vi "lfw_pairs.vi"(8 "error in (no error)":errorcluster caption="entrée d'erreur (pas d'erreur)", 11 "fetch_lfw_pairs":T2={"subset"="train", "funneled"=TRUE, "resize"=0.5, "color"=FALSE, "slice_"={"Cluster"={"height"=70, "width"=195}, "Cluster 2"={"height"=78, "width"=172}}, "download_if_missing"=TRUE, "Returns"="Data"}) -> (0 "error out":errorcluster, 3 "Data":T1)   [LabVIEW 2020]
doc: "Parameters :\n\n- subset : optional, default: ‘train’\nSelect the dataset to load: ‘train’ for the development training set, ‘test’ for the development test set, and ‘10_folds’ for the official evaluation set that is meant to be used with a 10-folds cross validation.\n\n- funneled : boolean, optional, default: True\nDownload and use the funneled variant of the dataset.\n\n- resize : float, optional, default 0.5\nRatio used to resize the each face picture.\n\n- color : boolean, optional, default False\nKeep the 3 RGB channels instead of averaging them to a single gray level channel. If color is True the shape of the data has one more dimension than the shape with color = False.\n\n- slice_ : optional\nProvide a custom 2D slice (height, width) to extract the ‘interesting’ part of the jpeg files and avoid use statistical correlation from the background\n\n- download_if_missing : optional, True by default\nIf False, raise a IOError if the data is not locally available instead of trying to download the data from the source site.\n\nReturns :\n\n- data : ndarray of shape (2200, 2, 62, 47). Shape depends on subset\nEach row has 2 face images corresponding to same or different person from the dataset containing 5749 people. Changing the slice_, resize or subset parameters will change the shape of the output.\n\n- target : numpy array of shape (2200,). Shape depends on subset.\nLabels associated to each pair of images. The two label values being different persons or the same person.\n\n\nEach picture is centered on a single face. The typical task is called Face Verification: given a pair of two pictures, a binary classifier must predict whether the two images are from the same person.\n\nBoth Face Verification and Face Recognition are tasks that are typically performed on the output of a model trained to perform Face Detection. The most popular model for Face Detection is called Viola-Jones and is implemented in the OpenCV library. The LFW faces were extracted by this face detector from various online websites.\n\nThe original images are 250 x 250 pixels, but the default slice and resize arguments reduce them to 62 x 47."
uses:
  lfw_pairs.lvclass
panel:
  out "lfw_pairs.lvclass":refnum<class "lfw_pairs.lvclass">
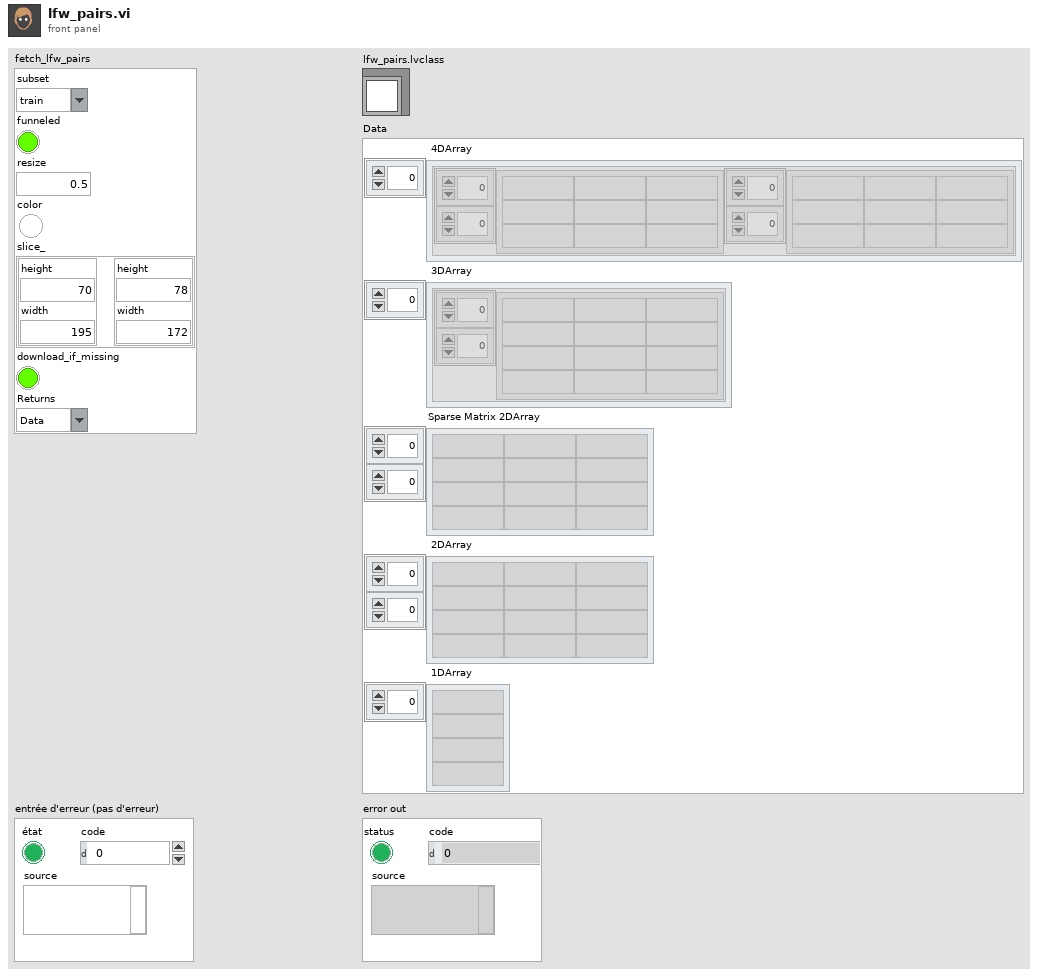
[diagram p1: front panel]
types:
  T1 = cluster{" 4DArray":cluster{"1":string[][], "2":string[][]}[], " 3DArray":cluster{"Tableau":string[][]}[], "Sparse Matrix 2DArray":string[][], " 2DArray":string[][], " 1DArray":string[]}
  T2 = cluster{"subset":string, "funneled":bool, "resize":dbl, "color":bool, "slice_":cluster{"Cluster":cluster{"height":u32, "width":u32}, "Cluster 2":cluster{"height":u32, "width":u32}}, "download_if_missing":bool, "Returns":string}
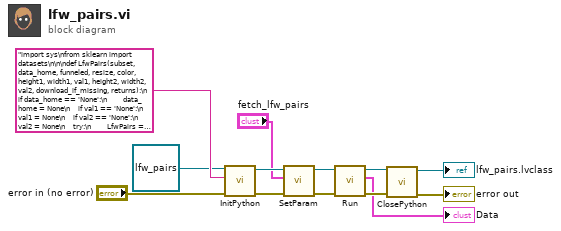
[diagram p0: block diagram]
diagram:
  n1 = call-dynamic "InitPython.vi"("error in (no error)"="error in (no error)", "Python Instruction"="import sys\nfrom sklearn import datasets\n\n\ndef LfwPairs(subset, data_home, funneled, resize, color, height1, width1, val1, height2, width2, val2, download_if_missing, returns):\n    if data_home == 'None':\n        data_home = None\n    if val1 == 'None':\n        val1 = None\n    if val2 == 'None':\n        val2 = None\n    try:\n        LfwPairs = datasets.fetch_lfw_pairs(subset, data_home, funneled, resize, color, (slice(height1, width1, val1), slice(height2, width2, val2)), download_if_missing)\n        if returns == 'Data': \n            data = LfwPairs['pairs'].tolist()\n            return str(data)\n        else :\n            data = LfwPairs['target'].tolist()\n            return str(data)\n    except:\n        erreur = sys.exc_info()\n        typerr = u\"%s\" % (erreur[0])\n        typerr = typerr[typerr.find(\"'\")+1:typerr.rfind(\"'\")]\n        msgerr = u\"%s\" % (erreur[1])\n        message = str('/!\\\\ {0} : {1}'. format(typerr,msgerr))\n        return message", "Scikit-learn en entrée"=refnum<class "lfw_pairs.lvclass"> refnum ("lfw_pairs.lvclass")) -> ("error out"=w8:errorcluster, "Scikit-learn en sortie"=w10:refnum<class "lfw_pairs.lvclass">)  [unwired: 7 in]
  n2 = call-dynamic "SetParam.vi"("error in (no error)"=w8, "fetch_lfw_pairs"="fetch_lfw_pairs", "lfw_pairs.lvclass"=w10) -> ("error out"=w6:errorcluster, "lfw_pairs.lvclass"=w7:refnum<class "lfw_pairs.lvclass">)  [unwired: 7 in]
  n3 = call-dynamic "Run.vi"("error in (no error)"=w6, "lfw_pairs.lvclass"=w7) -> ("error out"=w4:errorcluster, "Data"=→"Data":T1, "lfw_pairs.lvclass"=w5:refnum<class "lfw_pairs.lvclass">)  [unwired: 7 in]
  n4 = call-dynamic "ClosePython.vi"("error in (no error)"=w4, "Scikit-learn en entrée"=w5) -> ("error out"=→"error out":errorcluster, "Scikit-learn en sortie"=→"lfw_pairs.lvclass":refnum<class "lfw_pairs.lvclass">)  [unwired: 8 in]
